vi "Is Tagged Union.vi"(8 "Error In":errorcluster, 11 "Type in":variant) -> (0 "Error Out":errorcluster, 2 "Tagged Union?":bool, 3 "Type out":variant)   [LabVIEW 2015, in "Scripting.lvlib"]
uses:
  Scripting.lvlib
  <vilib>/Utility/Data Type/Type Definitions/Data Type.ctl
  <vilib>/Utility/Data Type/NI_Data Type.lvlib
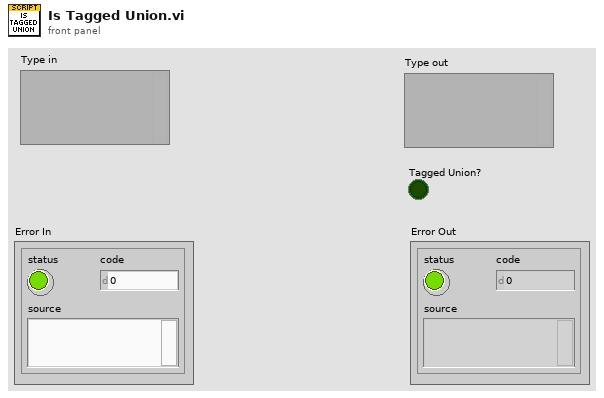
[diagram p1: front panel]
types:
  T1 = typedef "NI_Data Type.lvlib/Data Type.ctl" = enum8{"Invalid Type", "Void", "I8", "I16", "I32", "I64", "U8", "U16", "U32", "U64", "Single Float", "Double Float", "Extended Float", "Single Complex", "Double Complex", "Extended Complex", "Enum U8", "Enum U16", "Enum U32", "Enum U64", "Single Float With Unit", "Double Float With Unit", "Extended Float With Unit", "Single Complex with Unit", "Double Complex with Unit", "Extended Complex with Unit", "Boolean", "String", "Path", "Picture", "Tag", "Array", "Cluster", "Variant", "LV Variant", "Waveform", "Timestamp", "Digital Waveform", "Digital Data", "ExpressData", "Refnum", "External Data", "VI", "Poly VI", "LabVIEW Class Instance", "Fixed Point"}
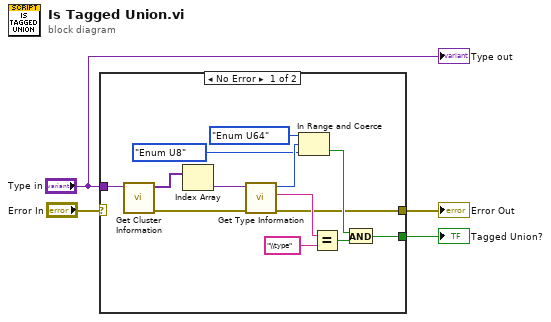
[diagram p0: block diagram]
diagram:
  n1 = case shown="No Error" "Error In" {
    selector: "Error In" -> [_ w18]
    tunnel: "Type in" -> [w17 _]
    tunnel: [w7 w18] -> w1
    tunnel: [w6 _] -> w3
    frame No Error {
      n2 = call <vilib>:"Get Cluster Information.vi"("Variant"=w17) -> ("error out"=w15:errorcluster, "Cluster Elements"=w16:variant[])  [unwired: 9 in]
      n3 = Index Array(array=w16) -> (element=w5:variant)  [unwired: 1 in]
      n4 = call <vilib>:"Get Type Information.vi"("error in (no error)"=w15, "Variant"=w5) -> ("error out"=w7:errorcluster, "Name"=w11:string, "Type"=w14:T1)  [unwired: 5 in, 2 out]
      n5 = In Range and Coerce(upper limit=Data_Type."Enum U64", x=w14, lower limit=Data_Type."Enum U8" ("upper limit")) -> (In Range?=w8:bool)  [unwired: 1 out]
      n6 = Equal?(x=w11, y="\\type") -> (x = y?=w9:bool)
      n7 = And(x=w8, y=w9) -> (x .and. y?=w6:bool)
    }
    frame Error {
    }
  }
  "Error Out" <- w1
  "Tagged Union?" <- w3
  "Type out" <- "Type in"
